vi "FreqOffset.vi"(0 "VISA IN":refnum<visa-resource-name>, 5 "error in":errorcluster) -> (14 "VISA Out":refnum<visa-resource-name>, 19 "error out":errorcluster)   [LabVIEW 2018, in "PNA-X.lvlib"]
uses:
  PNA-X.lvlib
panel:
  in  "Segment Function":enum16{"ADD", "DELETE"}(ring)
  in  "Source Port":i32=1
  in  "Stop":dbl=2000000000.0
  in  "Start":dbl=1000000000.0
  in  "Stimulus":bool=TRUE
  in  "Span":dbl=1000000000.0
  in  "Center":dbl=1500000000.0
  in  "Stop":dbl=2000000000.0
  in  "Start":dbl=1000000000.0
  in  "Npoints":i32=201
  in  "IF BW":dbl=10000.0
  in  "Power Level":dbl=-20.0
  in  "Points":i32=201
  in  "Segment":i32=1
  in  "Independent Power Levels? ON/OFF":bool
  in  "Independent IF BW? ON/OFF":bool
  in  "Independent Sweep Time? ON/OFF":bool
  in  "Segment Number - State? ON/OFF":bool=TRUE
  in  "Time":dbl=3.0
  in  "CW Frq.":dbl=5000000000.0
  in  "Sweep Time(sec)":dbl=3.0
  in  "CW Frq.":dbl=10000000000.0
  in  "Offset":dbl=1000000.0
  in  "Divisor":i32=1
  in  "Multiplier":i32=1
  in  "Couple Range to Primary Range ON/OFF":bool
  in  "Sweep Type":string(combo)="LINear"
  in  "Range number":i32=1
  in  "Frq. Offset ON/OFF":bool=TRUE
  in  "Channel":i32=1
  # "Un-Coupled and Primary Settings"
  # "Segment Sweep Properties"
  # "Linear and Log Properties"
  # "<-->"
  # "<-->"
  # "CW Time Properties"
  # "Power Sweep Properties"
  # "Coupled Settings"
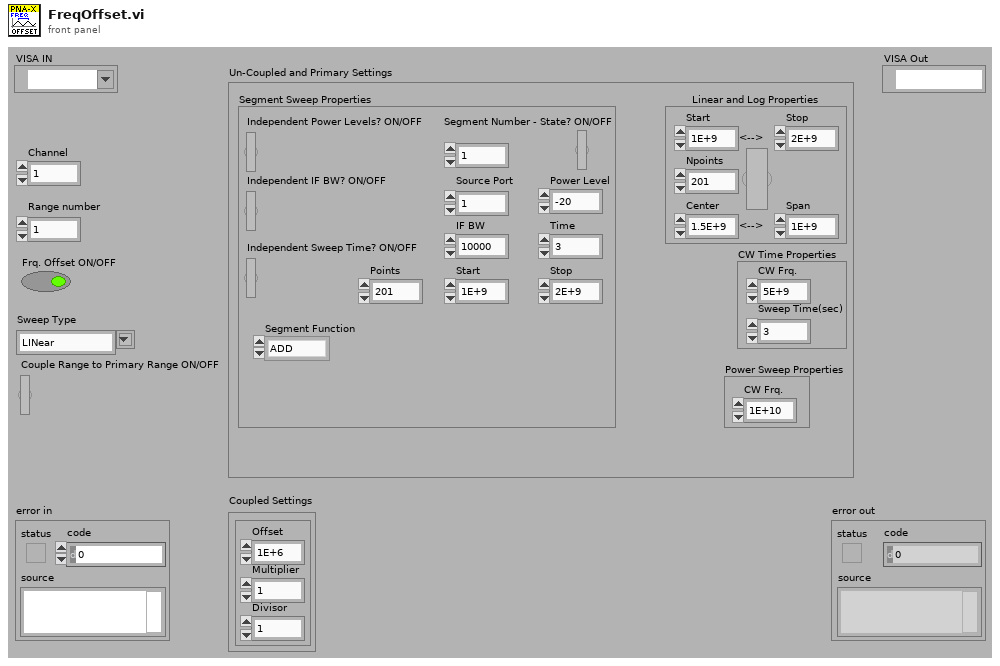
[diagram p1: front panel]
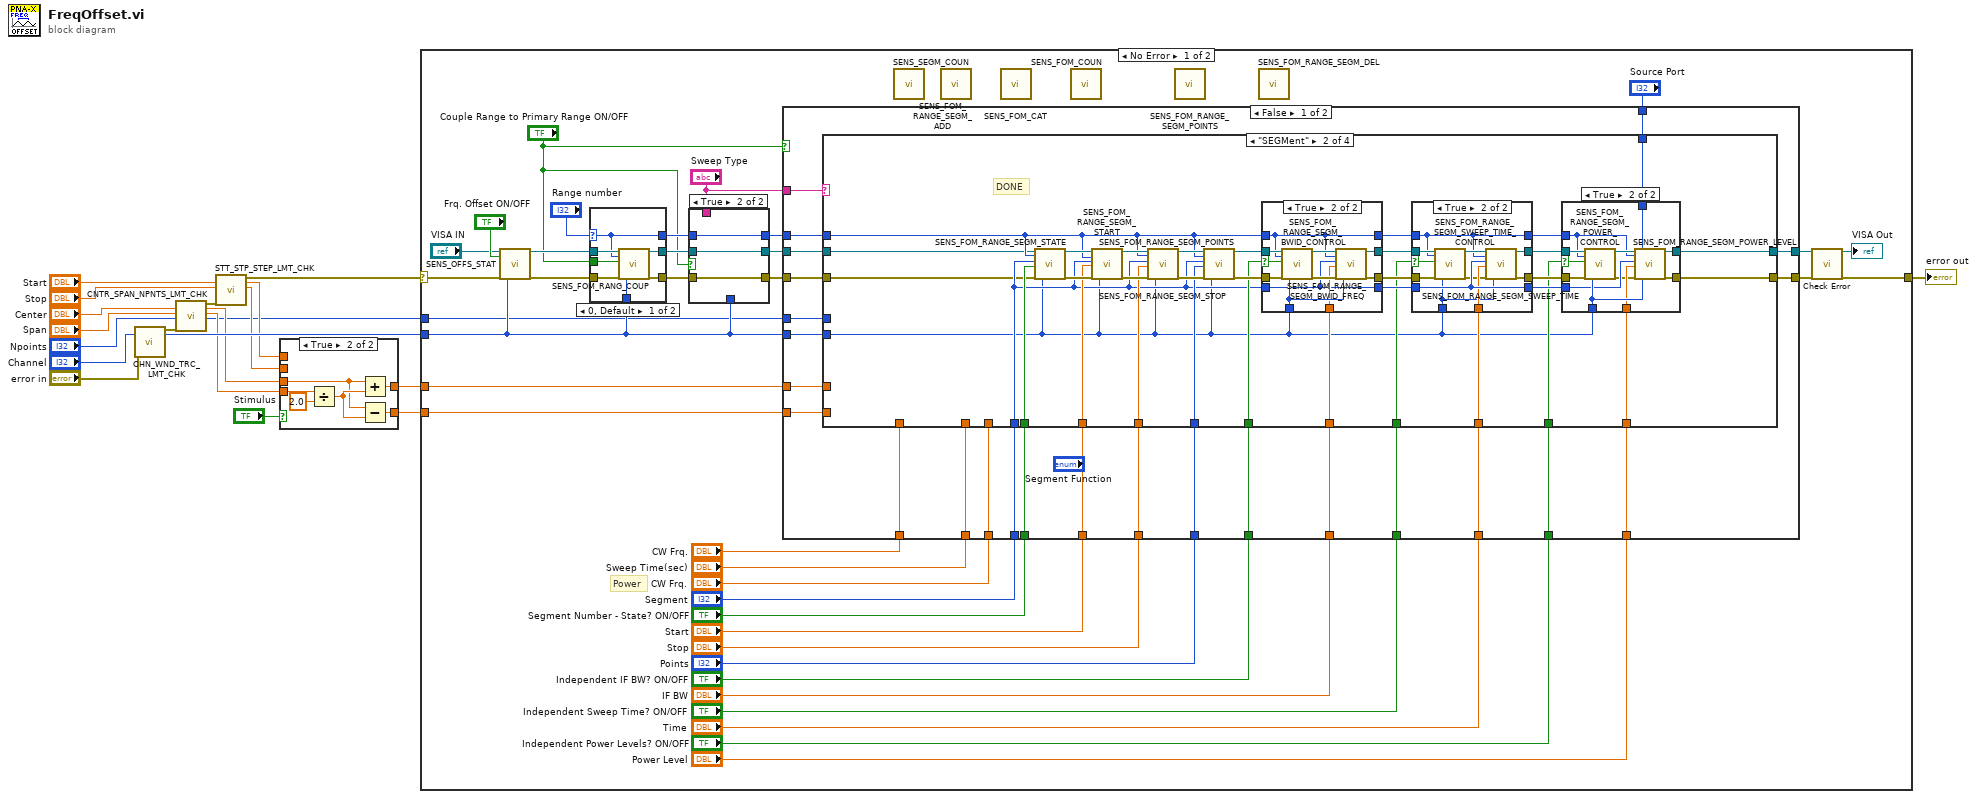
[diagram p0: block diagram]
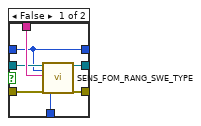
[diagram p3: hidden frame]
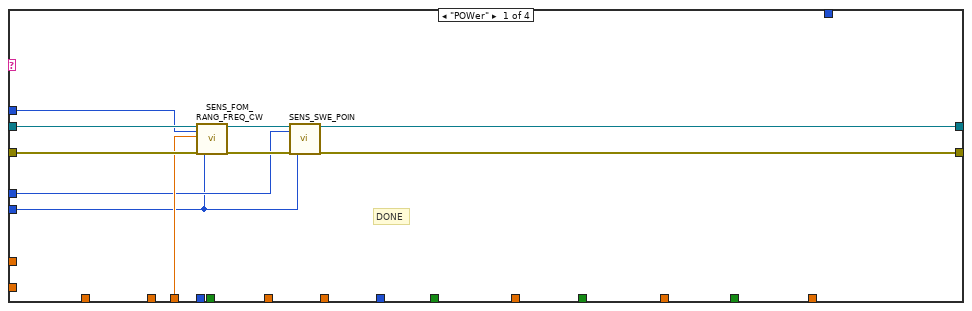
[diagram p5: hidden frame]
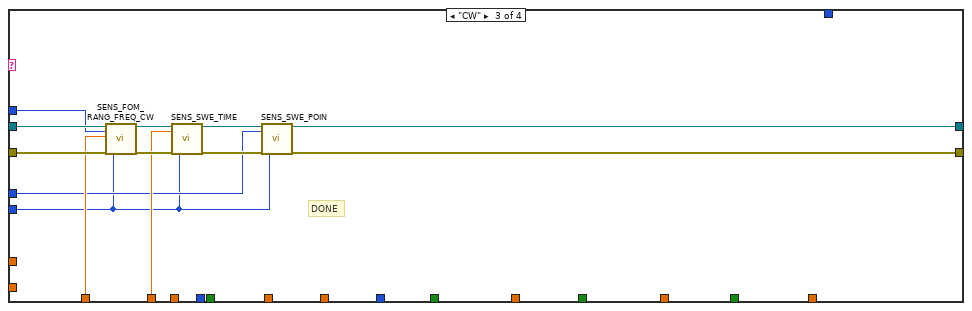
[diagram p9: hidden frame]
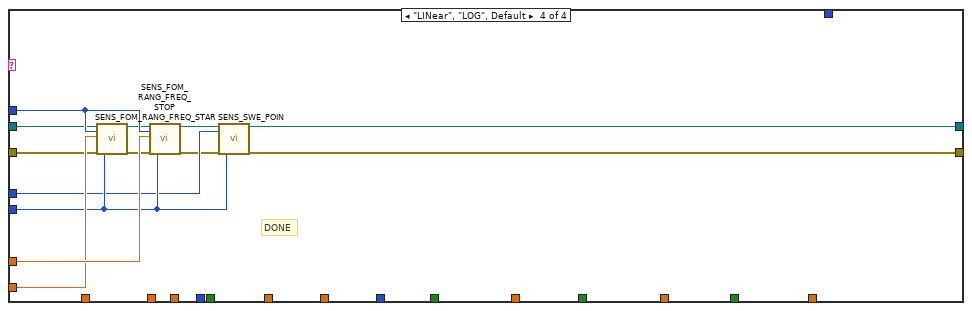
[diagram p10: hidden frame]
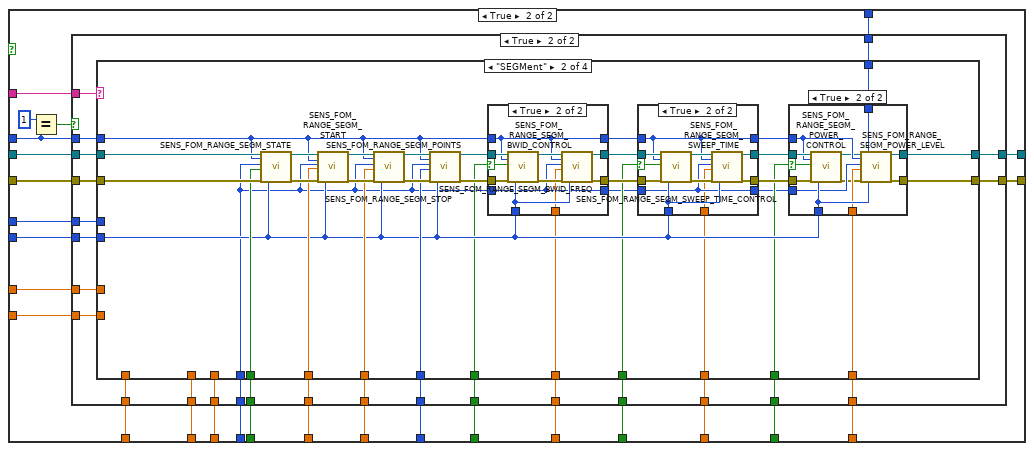
[diagram p11: hidden frame]
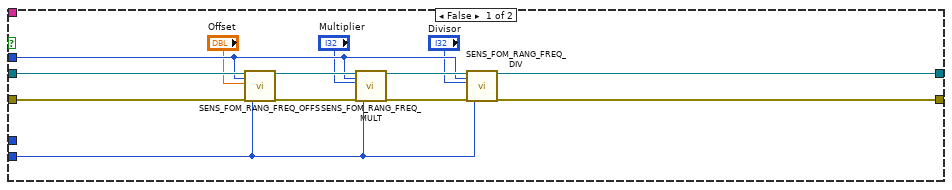
[diagram p12: hidden frame]
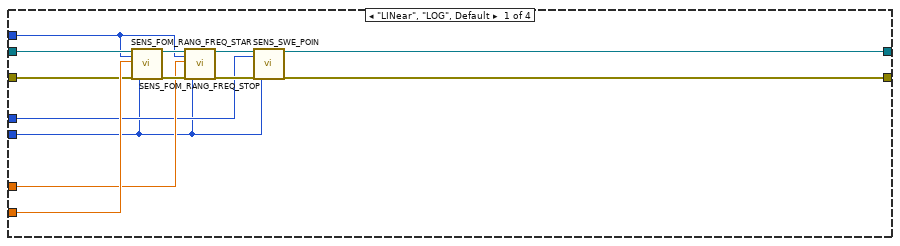
[diagram p13: hidden frame]
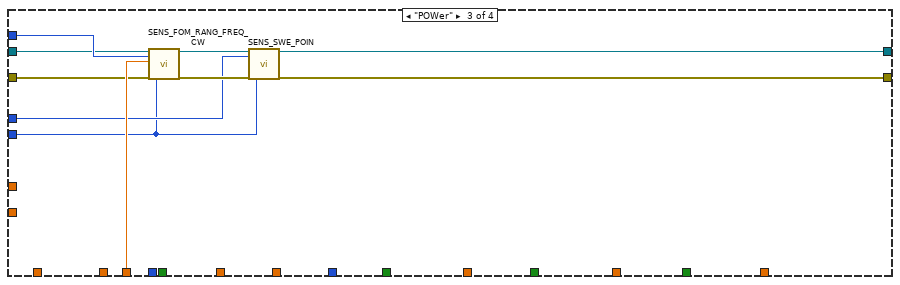
[diagram p17: hidden frame]
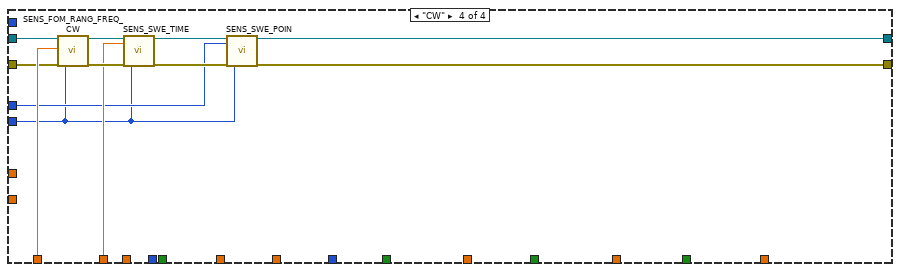
[diagram p18: hidden frame]
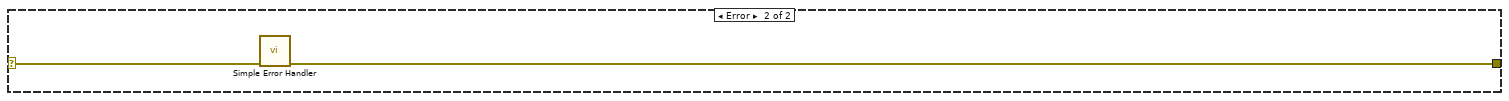
[diagram p19: hidden frame]
diagram:
  n1 = call "CHN_WND_TRC_LMT_CHK.vi"("Channel"="Channel", "error in"="error in") -> ("error out"=w20:errorcluster, "Channel"=w11:i32)  [unwired: 13 in, 3 out]
  n2 = call "CNTR_SPAN_NPNTS_LMT_CHK.vi"("Center"="Center", "Span"="Span", "Npoints"="Npoints", "error in"=w20) -> ("error out"=w14:errorcluster, "Center"=w7:dbl, "Span"=w6:dbl, "Npoints"=w1:i32)  [unwired: 12 in]
  n3 = call "STT_STP_STEP_LMT_CHK.vi"("Start"="Start", "Stop"="Stop", "error in"=w14) -> ("error out"=w13:errorcluster, "Start"=w4:dbl, "Stop"=w5:dbl)  [unwired: 13 in, 1 out]
  n4 = case shown="True" "Stimulus" {
    tunnel: w7 -> [_ w26]
    tunnel: w6 -> [_ w25]
    tunnel: [w22 w24] -> w2
    tunnel: w5 -> [w21 _]
    tunnel: w4 -> [w22 _]
    tunnel: [w21 w23] -> w3
    frame False {
    }
    frame True {
      n5 = Divide(x=w25, y=2.0) -> (x/y=w27:dbl)
      n6 = Add(x=w26, y=w27) -> (x+y=w24:dbl)
      n7 = Subtract(x=w26, y=w27) -> (x-y=w23:dbl)
    }
  }
  n8 = case shown="No Error" w13 {
    selector: w13 -> [w60 w404]
    tunnel: [w51 w403] -> w15
    tunnel: w11 -> [w55 _]
    tunnel: w2 -> [w65 _]
    tunnel: w3 -> [w64 _]
    tunnel: w1 -> [w50 _]
    frame No Error {
      # "Power"
      n9 = call "SENS_OFFS_STAT.vi"("VISA IN"="VISA IN", "Frq. Offset ON/OFF"="Frq. Offset ON/OFF", "error in"=w60, "Channel"=w55) -> ("VISA Out"=w57:refnum<visa-resource-name>, "error out"=w56:errorcluster)  [unwired: 14 in]
      n10 = case shown="0, Default" "Range number" {
        selector: "Range number" -> [w76 w85]
        tunnel: w57 -> [w82 w84]
        tunnel: w56 -> [w81 w83]
        tunnel: w55 -> [w80 _]
        tunnel: "Couple Range to Primary Range ON/OFF" -> [w79 _]
        tunnel: [w78 w83] -> w32
        tunnel: [w77 w84] -> w35
        tunnel: [w76 w85] -> w33
        frame 0, Default {
          n11 = call "SENS_FOM_RANG_COUP.vi"("VISA IN"=w82, "Range number"=w76, "Couple Range to Primary Range ON/OFF"=w79, "error in"=w81, "Channel"=w80) -> ("VISA Out"=w77:refnum<visa-resource-name>, "error out"=w78:errorcluster)  [unwired: 13 in]
        }
        frame 1 {
        }
      }
      n12 = case shown="True" "Couple Range to Primary Range ON/OFF" {
        tunnel: [w72 w74] -> w63
        tunnel: "Sweep Type" -> [w71 _]
        tunnel: [w70 w75] -> w58
        tunnel: w55 -> [w69 _]
        tunnel: w35 -> [w68 w75]
        tunnel: w33 -> [w66 w73]
        tunnel: w32 -> [w67 w74]
        tunnel: [w66 w73] -> w29
        frame False {
          n13 = call "SENS_FOM_RANG_SWE_TYPE.vi"("VISA IN"=w68, "Range number"=w66, "Sweep Type"=w71, "error in"=w67, "Channel"=w69) -> ("VISA Out"=w70:refnum<visa-resource-name>, "error out"=w72:errorcluster)  [unwired: 13 in]
        }
        frame True {
        }
      }
      n14 = case shown="False" "Couple Range to Primary Range ON/OFF" {
        tunnel: w65 -> [w110 w230]
        tunnel: w64 -> [w109 w231]
        tunnel: w63 -> [w108 w251]
        tunnel: "Sweep Type" -> [w107 w232]
        tunnel: w58 -> [w106 w249]
        tunnel: w55 -> [w105 w247]
        tunnel: w29 -> [w104 w235]
        tunnel: [w103 w248] -> w53
        tunnel: [w102 w250] -> w52
        tunnel: w50 -> [w101 w229]
        tunnel: "Segment Number - State? ON/OFF" -> [w88 w246]
        tunnel: "Segment" -> [w87 w245]
        tunnel: "Start" -> [w89 w244]
        tunnel: "Stop" -> [w90 w243]
        tunnel: "Points" -> [w91 w242]
        tunnel: "Independent IF BW? ON/OFF" -> [w92 w241]
        tunnel: "Independent Sweep Time? ON/OFF" -> [w94 w240]
        tunnel: "Independent Power Levels? ON/OFF" -> [w96 w239]
        tunnel: "IF BW" -> [w93 w238]
        tunnel: "Time" -> [w95 w237]
        tunnel: "Power Level" -> [w97 w236]
        tunnel: "CW Frq." -> [w100 w228]
        tunnel: "CW Frq." -> [w99 w227]
        tunnel: "Sweep Time(sec)" -> [w98 w226]
        tunnel: "Source Port" -> [w86 w225]
        frame False {
          n15 = case shown="\"SEGMent\"" w107 {
            tunnel: [w111 w122 w199 w220] -> w102
            tunnel: w108 -> [w119 w124 w209 w214]
            tunnel: w105 -> [w113 w127 w201 w219]
            tunnel: w110 -> [_ _ _ w224]
            tunnel: w109 -> [_ _ _ w223]
            tunnel: w104 -> [w118 w126 w207 w222]
            tunnel: w106 -> [w120 w125 w211 w217]
            tunnel: [w112 w123 w200 w221] -> w103
            tunnel: w101 -> [w114 _ w202 w218]
            tunnel: w100 -> [w117 _ _ _]
            tunnel: w99 -> [_ _ w206 _]
            tunnel: w98 -> [_ _ w205 _]
            tunnel: w97 -> [_ w138 _ _]
            tunnel: w96 -> [_ w137 _ _]
            tunnel: w95 -> [_ w136 _ _]
            tunnel: w94 -> [_ w135 _ _]
            tunnel: w93 -> [_ w134 _ _]
            tunnel: w92 -> [_ w133 _ _]
            tunnel: w91 -> [_ w132 _ _]
            tunnel: w90 -> [_ w131 _ _]
            tunnel: w89 -> [_ w130 _ _]
            tunnel: w88 -> [_ w129 _ _]
            tunnel: w87 -> [_ w128 _ _]
            tunnel: w86 -> [_ w121 _ _]
            frame "POWer" {
              # "DONE"
              n16 = call "SENS_FOM_RANG_FREQ_CW.vi"("VISA IN"=w120, "Range number"=w118, "CW Frq.(Hz)"=w117, "error in"=w119, "Channel"=w113) -> ("VISA Out"=w116:refnum<visa-resource-name>, "error out"=w115:errorcluster)  [unwired: 13 in]
              n17 = call "SENS_SWE_POIN.vi"("VISA IN"=w116, "Sweep Points"=w114, "error in"=w115, "Channel"=w113) -> ("VISA Out"=w112:refnum<visa-resource-name>, "error out"=w111:errorcluster)  [unwired: 14 in]
            }
            frame "SEGMent" {
              # "DONE"
              n18 = call "SENS_FOM_RANGE_SEGM_STATE.vi"("VISA IN"=w125, "Range"=w126, "Segment"=w128, "ON/OFF"=w129, "error in"=w124, "Channel"=w127) -> ("VISA Out"=w151:refnum<visa-resource-name>, "error out"=w154:errorcluster)  [unwired: 12 in]
              n19 = call "SENS_FOM_RANGE_SEGM_START.vi"("VISA IN"=w151, "Range"=w126, "Segment"=w128, "Start Frequency"=w130, "error in"=w154, "Channel"=w127) -> ("VISA Out"=w150:refnum<visa-resource-name>, "error out"=w153:errorcluster)  [unwired: 12 in]
              n20 = call "SENS_FOM_RANGE_SEGM_STOP.vi"("VISA IN"=w150, "Range"=w126, "Segment"=w128, "Stop Frequency"=w131, "error in"=w153, "Channel"=w127) -> ("VISA Out"=w149:refnum<visa-resource-name>, "error out"=w152:errorcluster)  [unwired: 12 in]
              n21 = call "SENS_FOM_RANGE_SEGM_POINTS.vi"("VISA IN"=w149, "Range"=w126, "Segment"=w128, "Points"=w132, "error in"=w152, "Channel"=w127) -> ("VISA Out"=w145:refnum<visa-resource-name>, "error out"=w146:errorcluster)  [unwired: 12 in]
              n22 = case shown="True" w133 {
                selector: w133 -> [_ w190]
                tunnel: w126 -> [w187 w191]
                tunnel: [w187 w191] -> w148
                tunnel: w127 -> [_ w196]
                tunnel: w146 -> [w186 w195]
                tunnel: w145 -> [w185 w194]
                tunnel: [w186 w193] -> w144
                tunnel: [w185 w192] -> w142
                tunnel: w134 -> [_ w189]
                tunnel: w128 -> [w184 w188]
                tunnel: [w184 w188] -> w140
                frame False {
                }
                frame True {
                  n23 = call "SENS_FOM_RANGE_SEGM_BWID_CONTROL.vi"("VISA IN"=w194, "Range"=w191, "Enable BWID? ON/OFF"=w190, "error in"=w195, "Channel"=w196) -> ("VISA Out"=w198:refnum<visa-resource-name>, "error out"=w197:errorcluster)  [unwired: 13 in]
                  n24 = call "SENS_FOM_RANGE_SEGM_BWID_FREQ.vi"("VISA IN"=w198, "Range"=w191, "Segment"=w188, "IF BW(Hz)"=w189, "error in"=w197, "Channel"=w196) -> ("VISA Out"=w192:refnum<visa-resource-name>, "error out"=w193:errorcluster)  [unwired: 12 in]
                }
              }
              n25 = case shown="True" w135 {
                selector: w135 -> [_ w174]
                tunnel: w148 -> [w172 w173]
                tunnel: [w172 w173] -> w147
                tunnel: w127 -> [_ w175]
                tunnel: w144 -> [w171 w177]
                tunnel: [w171 w183] -> w143
                tunnel: w142 -> [w170 w179]
                tunnel: [w170 w182] -> w141
                tunnel: w140 -> [w169 w181]
                tunnel: [w169 w181] -> w139
                tunnel: w136 -> [_ w180]
                frame False {
                }
                frame True {
                  n26 = call "SENS_FOM_RANGE_SEGM_SWEEP_TIME_CONTROL.vi"("VISA IN"=w179, "Range"=w173, "Enable Sweep Time? ON/OFF"=w174, "error in"=w177, "Channel"=w175) -> ("VISA Out"=w178:refnum<visa-resource-name>, "error out"=w176:errorcluster)  [unwired: 13 in]
                  n27 = call "SENS_FOM_RANGE_SEGM_SWEEP_TIME.vi"("VISA IN"=w178, "Range"=w173, "Segment"=w181, "Sweep Time(sec)"=w180, "error in"=w176, "Channel"=w175) -> ("VISA Out"=w182:refnum<visa-resource-name>, "error out"=w183:errorcluster)  [unwired: 12 in]
                }
              }
              n28 = case shown="True" w137 {
                selector: w137 -> [_ w161]
                tunnel: [w156 w168] -> w122
                tunnel: [w155 w167] -> w123
                tunnel: w147 -> [_ w162]
                tunnel: w127 -> [_ w166]
                tunnel: w143 -> [w156 w165]
                tunnel: w141 -> [w155 w164]
                tunnel: w139 -> [_ w160]
                tunnel: w138 -> [_ w159]
                tunnel: w121 -> [_ w157]
                frame False {
                }
                frame True {
                  n29 = call "SENS_FOM_RANGE_SEGM_POWER_CONTROL.vi"("VISA IN"=w164, "Range"=w162, "Enable Power Level? ON/OFF"=w161, "error in"=w165, "Channel"=w166) -> ("VISA Out"=w163:refnum<visa-resource-name>, "error out"=w158:errorcluster)  [unwired: 13 in]
                  n30 = call "SENS_FOM_RANGE_SEGM_POWER_LEVEL.vi"("VISA IN"=w163, "Range"=w162, "Segment"=w160, "Power Level"=w159, "error in"=w158, "Source Port"=w157, "Channel"=w166) -> ("VISA Out"=w167:refnum<visa-resource-name>, "error out"=w168:errorcluster)  [unwired: 11 in]
                }
              }
            }
            frame "CW" {
              # "DONE"
              n31 = call "SENS_FOM_RANG_FREQ_CW.vi"("VISA IN"=w211, "Range number"=w207, "CW Frq.(Hz)"=w206, "error in"=w209, "Channel"=w201) -> ("VISA Out"=w210:refnum<visa-resource-name>, "error out"=w208:errorcluster)  [unwired: 13 in]
              n32 = call "SENS_SWE_TIME.vi"("VISA IN"=w210, "Sweep Time(sec)"=w205, "error in"=w208, "Channel"=w201) -> ("VISA Out"=w204:refnum<visa-resource-name>, "error out"=w203:errorcluster)  [unwired: 14 in]
              n33 = call "SENS_SWE_POIN.vi"("VISA IN"=w204, "Sweep Points"=w202, "error in"=w203, "Channel"=w201) -> ("VISA Out"=w200:refnum<visa-resource-name>, "error out"=w199:errorcluster)  [unwired: 14 in]
            }
            frame "LINear", "LOG", Default {
              # "DONE"
              n34 = call "SENS_FOM_RANG_FREQ_STAR.vi"("VISA IN"=w217, "Range number"=w222, "Frq. Start"=w223, "error in"=w214, "Channel"=w219) -> ("VISA Out"=w216:refnum<visa-resource-name>, "error out"=w213:errorcluster)  [unwired: 13 in]
              n35 = call "SENS_FOM_RANG_FREQ_STOP.vi"("VISA IN"=w216, "Range number"=w222, "Frq. Stop"=w224, "error in"=w213, "Channel"=w219) -> ("VISA Out"=w215:refnum<visa-resource-name>, "error out"=w212:errorcluster)  [unwired: 13 in]
              n36 = call "SENS_SWE_POIN.vi"("VISA IN"=w215, "Sweep Points"=w218, "error in"=w212, "Channel"=w219) -> ("VISA Out"=w221:refnum<visa-resource-name>, "error out"=w220:errorcluster)  [unwired: 14 in]
            }
          }
        }
        frame True {
          n37 = Equal?(x=1, y=w235) -> (x = y?=w233:bool)
          n38 = case shown="True" w233 {
            tunnel: w251 -> [w264 w289]
            tunnel: [w261 w288] -> w250
            tunnel: w249 -> [w260 w287]
            tunnel: [w257 w286] -> w248
            tunnel: w235 -> [w256 w285]
            tunnel: w247 -> [w255 w280]
            tunnel: w246 -> [_ w284]
            tunnel: w245 -> [_ w275]
            tunnel: w244 -> [_ w283]
            tunnel: w243 -> [_ w282]
            tunnel: w242 -> [_ w281]
            tunnel: w241 -> [_ w279]
            tunnel: w240 -> [_ w278]
            tunnel: w239 -> [_ w277]
            tunnel: w238 -> [_ w276]
            tunnel: w237 -> [_ w274]
            tunnel: w236 -> [_ w273]
            tunnel: w232 -> [_ w272]
            tunnel: w231 -> [_ w271]
            tunnel: w230 -> [_ w270]
            tunnel: w229 -> [_ w269]
            tunnel: w228 -> [_ w268]
            tunnel: w227 -> [_ w267]
            tunnel: w226 -> [_ w266]
            tunnel: w225 -> [_ w265]
            frame False {
              n39 = call "SENS_FOM_RANG_FREQ_OFFS.vi"("VISA IN"=w260, "Range number"=w256, "Offset Value"="Offset", "error in"=w264, "Channel"=w255) -> ("VISA Out"=w259:refnum<visa-resource-name>, "error out"=w263:errorcluster)  [unwired: 13 in]
              n40 = call "SENS_FOM_RANG_FREQ_MULT.vi"("VISA IN"=w259, "Range number"=w256, "Multiplier Value"="Multiplier", "error in"=w263, "Channel"=w255) -> ("VISA Out"=w258:refnum<visa-resource-name>, "error out"=w262:errorcluster)  [unwired: 13 in]
              n41 = call "SENS_FOM_RANG_FREQ_DIV.vi"("VISA IN"=w258, "Range number"=w256, "Divisor Value"="Divisor", "error in"=w262, "Channel"=w255) -> ("VISA Out"=w257:refnum<visa-resource-name>, "error out"=w261:errorcluster)  [unwired: 13 in]
            }
            frame True {
              n42 = case shown="\"SEGMent\"" w272 {
                tunnel: w289 -> [w294 w336 w388 w398]
                tunnel: [w293 w332 w383 w394] -> w288
                tunnel: w287 -> [w292 w331 w387 w397]
                tunnel: [w291 w327 w384 w393] -> w286
                tunnel: w285 -> [w290 w326 w389 _]
                tunnel: w284 -> [_ w325 _ _]
                tunnel: w283 -> [_ w324 _ _]
                tunnel: w282 -> [_ w323 _ _]
                tunnel: w281 -> [_ w322 _ _]
                tunnel: w280 -> [w295 w319 w381 w391]
                tunnel: w279 -> [_ w312 _ _]
                tunnel: w278 -> [_ w311 _ _]
                tunnel: w277 -> [_ w310 _ _]
                tunnel: w276 -> [_ w309 _ _]
                tunnel: w275 -> [_ w308 _ _]
                tunnel: w274 -> [_ w305 _ _]
                tunnel: w273 -> [_ w304 _ _]
                tunnel: w271 -> [w298 _ _ _]
                tunnel: w270 -> [w297 _ _ _]
                tunnel: w269 -> [w296 _ w382 w392]
                tunnel: w268 -> [_ _ w390 _]
                tunnel: w267 -> [_ _ _ w400]
                tunnel: w266 -> [_ _ _ w399]
                tunnel: w265 -> [_ w303 _ _]
                frame "LINear", "LOG", Default {
                  n43 = call "SENS_FOM_RANG_FREQ_STAR.vi"("VISA IN"=w292, "Range number"=w290, "Frq. Start"=w298, "error in"=w294, "Channel"=w295) -> ("VISA Out"=w302:refnum<visa-resource-name>, "error out"=w301:errorcluster)  [unwired: 13 in]
                  n44 = call "SENS_FOM_RANG_FREQ_STOP.vi"("VISA IN"=w302, "Range number"=w290, "Frq. Stop"=w297, "error in"=w301, "Channel"=w295) -> ("VISA Out"=w300:refnum<visa-resource-name>, "error out"=w299:errorcluster)  [unwired: 13 in]
                  n45 = call "SENS_SWE_POIN.vi"("VISA IN"=w300, "Sweep Points"=w296, "error in"=w299, "Channel"=w295) -> ("VISA Out"=w291:refnum<visa-resource-name>, "error out"=w293:errorcluster)  [unwired: 14 in]
                }
                frame "SEGMent" {
                  n46 = call "SENS_FOM_RANGE_SEGM_STATE.vi"("VISA IN"=w331, "Range"=w326, "Segment"=w308, "ON/OFF"=w325, "error in"=w336, "Channel"=w319) -> ("VISA Out"=w330:refnum<visa-resource-name>, "error out"=w335:errorcluster)  [unwired: 12 in]
                  n47 = call "SENS_FOM_RANGE_SEGM_START.vi"("VISA IN"=w330, "Range"=w326, "Segment"=w308, "Start Frequency"=w324, "error in"=w335, "Channel"=w319) -> ("VISA Out"=w329:refnum<visa-resource-name>, "error out"=w334:errorcluster)  [unwired: 12 in]
                  n48 = call "SENS_FOM_RANGE_SEGM_STOP.vi"("VISA IN"=w329, "Range"=w326, "Segment"=w308, "Stop Frequency"=w323, "error in"=w334, "Channel"=w319) -> ("VISA Out"=w328:refnum<visa-resource-name>, "error out"=w333:errorcluster)  [unwired: 12 in]
                  n49 = call "SENS_FOM_RANGE_SEGM_POINTS.vi"("VISA IN"=w328, "Range"=w326, "Segment"=w308, "Points"=w322, "error in"=w333, "Channel"=w319) -> ("VISA Out"=w317:refnum<visa-resource-name>, "error out"=w318:errorcluster)  [unwired: 12 in]
                  n50 = case shown="True" w312 {
                    selector: w312 -> [_ w372]
                    tunnel: w326 -> [w369 w373]
                    tunnel: [w369 w373] -> w321
                    tunnel: w319 -> [_ w378]
                    tunnel: w318 -> [w368 w377]
                    tunnel: w317 -> [w367 w376]
                    tunnel: [w368 w375] -> w316
                    tunnel: [w367 w374] -> w314
                    tunnel: w309 -> [_ w371]
                    tunnel: w308 -> [w366 w370]
                    tunnel: [w366 w370] -> w307
                    frame False {
                    }
                    frame True {
                      n51 = call "SENS_FOM_RANGE_SEGM_BWID_CONTROL.vi"("VISA IN"=w376, "Range"=w373, "Enable BWID? ON/OFF"=w372, "error in"=w377, "Channel"=w378) -> ("VISA Out"=w380:refnum<visa-resource-name>, "error out"=w379:errorcluster)  [unwired: 13 in]
                      n52 = call "SENS_FOM_RANGE_SEGM_BWID_FREQ.vi"("VISA IN"=w380, "Range"=w373, "Segment"=w370, "IF BW(Hz)"=w371, "error in"=w379, "Channel"=w378) -> ("VISA Out"=w374:refnum<visa-resource-name>, "error out"=w375:errorcluster)  [unwired: 12 in]
                    }
                  }
                  n53 = case shown="True" w311 {
                    selector: w311 -> [_ w357]
                    tunnel: w321 -> [w354 w358]
                    tunnel: [w354 w358] -> w320
                    tunnel: w319 -> [_ w365]
                    tunnel: w316 -> [w353 w364]
                    tunnel: [w353 w362] -> w315
                    tunnel: w314 -> [w352 w361]
                    tunnel: [w352 w359] -> w313
                    tunnel: w307 -> [w351 w356]
                    tunnel: [w351 w356] -> w306
                    tunnel: w305 -> [_ w355]
                    frame False {
                    }
                    frame True {
                      n54 = call "SENS_FOM_RANGE_SEGM_SWEEP_TIME_CONTROL.vi"("VISA IN"=w361, "Range"=w358, "Enable Sweep Time? ON/OFF"=w357, "error in"=w364, "Channel"=w365) -> ("VISA Out"=w360:refnum<visa-resource-name>, "error out"=w363:errorcluster)  [unwired: 13 in]
                      n55 = call "SENS_FOM_RANGE_SEGM_SWEEP_TIME.vi"("VISA IN"=w360, "Range"=w358, "Segment"=w356, "Sweep Time(sec)"=w355, "error in"=w363, "Channel"=w365) -> ("VISA Out"=w359:refnum<visa-resource-name>, "error out"=w362:errorcluster)  [unwired: 12 in]
                    }
                  }
                  n56 = case shown="True" w310 {
                    selector: w310 -> [_ w344]
                    tunnel: [w338 w350] -> w332
                    tunnel: [w337 w349] -> w327
                    tunnel: w320 -> [_ w345]
                    tunnel: w319 -> [_ w348]
                    tunnel: w315 -> [w338 w347]
                    tunnel: w313 -> [w337 w346]
                    tunnel: w306 -> [_ w343]
                    tunnel: w304 -> [_ w342]
                    tunnel: w303 -> [_ w339]
                    frame False {
                    }
                    frame True {
                      n57 = call "SENS_FOM_RANGE_SEGM_POWER_CONTROL.vi"("VISA IN"=w346, "Range"=w345, "Enable Power Level? ON/OFF"=w344, "error in"=w347, "Channel"=w348) -> ("VISA Out"=w340:refnum<visa-resource-name>, "error out"=w341:errorcluster)  [unwired: 13 in]
                      n58 = call "SENS_FOM_RANGE_SEGM_POWER_LEVEL.vi"("VISA IN"=w340, "Range"=w345, "Segment"=w343, "Power Level"=w342, "error in"=w341, "Source Port"=w339, "Channel"=w348) -> ("VISA Out"=w349:refnum<visa-resource-name>, "error out"=w350:errorcluster)  [unwired: 11 in]
                    }
                  }
                }
                frame "POWer" {
                  n59 = call "SENS_FOM_RANG_FREQ_CW.vi"("VISA IN"=w387, "Range number"=w389, "CW Frq.(Hz)"=w390, "error in"=w388, "Channel"=w381) -> ("VISA Out"=w386:refnum<visa-resource-name>, "error out"=w385:errorcluster)  [unwired: 13 in]
                  n60 = call "SENS_SWE_POIN.vi"("VISA IN"=w386, "Sweep Points"=w382, "error in"=w385, "Channel"=w381) -> ("VISA Out"=w384:refnum<visa-resource-name>, "error out"=w383:errorcluster)  [unwired: 14 in]
                }
                frame "CW" {
                  n61 = call "SENS_FOM_RANG_FREQ_CW.vi"("VISA IN"=w397, "CW Frq.(Hz)"=w400, "error in"=w398, "Channel"=w391) -> ("VISA Out"=w402:refnum<visa-resource-name>, "error out"=w401:errorcluster)  [unwired: 14 in]
                  n62 = call "SENS_SWE_TIME.vi"("VISA IN"=w402, "Sweep Time(sec)"=w399, "error in"=w401, "Channel"=w391) -> ("VISA Out"=w396:refnum<visa-resource-name>, "error out"=w395:errorcluster)  [unwired: 14 in]
                  n63 = call "SENS_SWE_POIN.vi"("VISA IN"=w396, "Sweep Points"=w392, "error in"=w395, "Channel"=w391) -> ("VISA Out"=w393:refnum<visa-resource-name>, "error out"=w394:errorcluster)  [unwired: 14 in]
                }
              }
            }
          }
        }
      }
      n64 = call "SENS_SEGM_COUN.vi"() -> ()  [unwired: 17 in, 3 out]
      n65 = call "SENS_FOM_RANGE_SEGM_ADD.vi"() -> ()  [unwired: 18 in, 2 out]
      n66 = call "SENS_FOM_CAT.vi"() -> ()  [unwired: 17 in, 3 out]
      n67 = call "SENS_FOM_COUN.vi"() -> ()  [unwired: 17 in, 3 out]
      n68 = call "SENS_FOM_RANGE_SEGM_POINTS.vi"() -> ()  [unwired: 18 in, 2 out]
      n69 = call "SENS_FOM_RANGE_SEGM_DEL.vi"() -> ()  [unwired: 18 in, 2 out]
      n70 = call "Check Error.vi"("VISA Resource Name"=w53, "error in (no error)"=w52) -> ("dup VISA session"=→"VISA Out":refnum<visa-resource-name>, "error out"=w51:errorcluster)  [unwired: 16 in]
    }
    frame Error {
      n71 = call <vilib>:"Simple Error Handler.vi"("error in (no error)"=w404) -> ("error out"=w403:errorcluster)  [unwired: 4 in, 4 out]
    }
  }
  "error out" <- w15
